vi "Notify.vi"(0 "reference in":refnum<class "Subject.lvclass">, 5 "error in (no error)":errorcluster) -> (14 "reference out":refnum<class "Subject.lvclass">, 19 "error out":errorcluster)   [LabVIEW 2013, in "Subject.lvclass"]
uses:
  Subject.lvclass
  ObServer_class/ObServer.lvclass
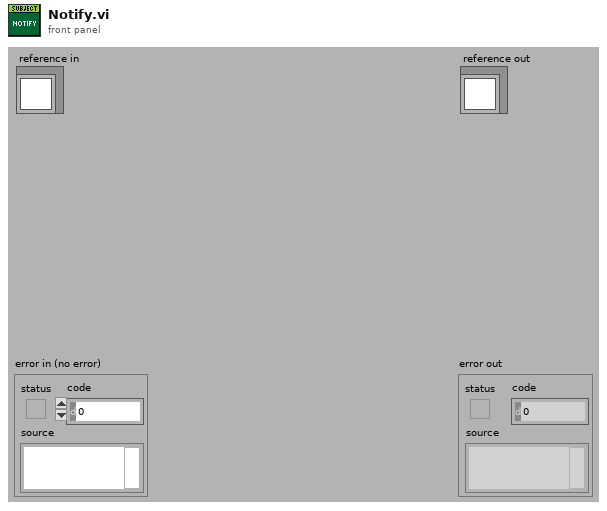
[diagram p1: front panel]
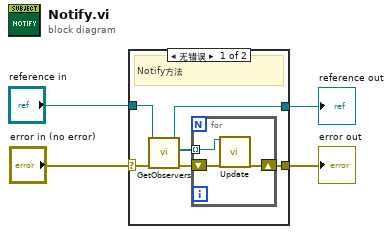
[diagram p0: block diagram]
diagram:
  n1 = case shown="无错误" "error in (no error)" {
    selector: "error in (no error)" -> [w6 w15]
    tunnel: [w7 w15] -> w3
    tunnel: [w9 w14] -> w1
    tunnel: "reference in" -> [w10 w14]
    frame No Error {
      # "Notify方法"
      n2 = call-dynamic "GetObservers.vi"("error in (no error)"=w6, "reference in"=w10) -> ("error out"=w5:errorcluster, "Observers"=w8:refnum<class "ObServer.lvclass">[], "reference out"=w9:refnum<class "Subject.lvclass">)  [unwired: 7 in]
      n3 = for {
        tunnel: w8 -> [w13] mode=indexing
        shift-right: [w11] -> w7
        shift-left: w5 -> [w12]
        n4 = call-dynamic "Update.vi"("reference in"=w13, "error in (no error)"=w12) -> ("error out"=w11:errorcluster)  [unwired: 16 in, 1 out]
      }
    }
    frame Error {
    }
  }
  "error out" <- w3
  "reference out" <- w1
